vi "写入缓存子集.vi"(8 "error in (no error)":errorcluster caption="错误输入（无错误）", 10 "缓存子集":cluster{"行":i32, "列":i32}[](array[cluster]), 11 "程序输入":refnum<class "程序.lvclass">) -> (0 "error out":errorcluster caption="错误输出", 3 "程序输出":refnum<class "程序.lvclass">)   [LabVIEW 2018, in "程序.lvclass"]
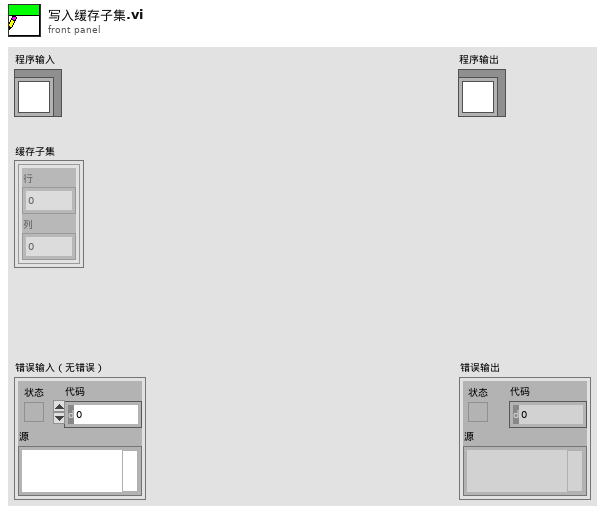
[diagram p1: front panel]
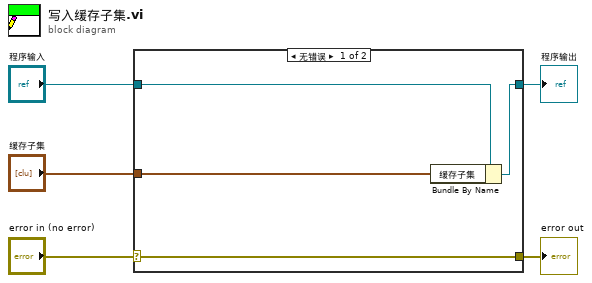
[diagram p0: block diagram]
diagram:
  n1 = case shown="无错误" "error in (no error)" {
    selector: "error in (no error)" -> [w9 w10]
    tunnel: [w9 w10] -> w4
    tunnel: [w7 w11] -> w2
    tunnel: "程序输入" -> [w8 w11]
    tunnel: "缓存子集" -> [w6 _]
    frame No Error {
      n2 = Bundle By Name(cluster=w8, "缓存子集"=w6) -> (w7:refnum<class "程序.lvclass">)
    }
    frame Error {
    }
  }
  "error out" <- w4
  "程序输出" <- w2
